vi "write_to_file.vi"(5 "y data precision":i16, 6 "x data precision":i16, 7 "y data":dbl, 8 "x data":dbl, 10 "refnum":refnum<file>) -> ()   [LabVIEW 2012]
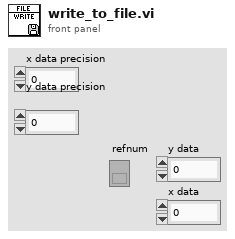
[diagram p1: front panel]
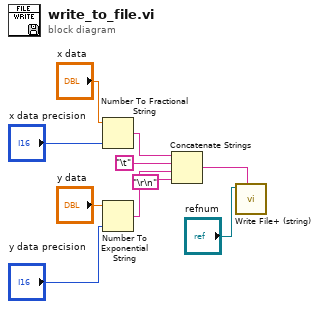
[diagram p0: block diagram]
diagram:
  n1 = Number To Fractional String(number="x data", precision (6)="x data precision") -> (F-format string=w8:string)  [unwired: 2 in]
  n2 = Number To Exponential String(number="y data", precision (6)="y data precision") -> (E-format string=w7:string)  [unwired: 2 in]
  n3 = Concatenate Strings(w8, "\t", w7, "\r\n") -> (w9:string)
  n4 = call <vilib>:"Write File+ (string).vi"("string"=w9, "refnum"="refnum") -> ()  [unwired: 5 in, 3 out]
